vi "1.1.vi"() -> ()   [LabVIEW 2020]
panel:
  in  "MODO 6":bool
  out "6":bool
  in  "MODO 5":bool
  out "5":bool
  in  "MODO 4":bool
  out "4":bool
  in  "MODO 3":bool
  out "3":bool
  in  "MODO 2":bool
  out "2":bool
  in  "MODO 1":bool
  out "1":bool
  # "SWITCH WHEN PRESSED: ESTE MODO MECANICO CAMBIA DE VALORA CADA QUE\nES PRESIONADO"
  # "SWITCH WHEN RELEASED: ESTE MODO CAMBIA CUANDO SE DEJA DE PRESIONAR"
  # "SWITCH UNTIL RELEASEDESTE MODO CAMBIA CUANDO SE PRESIONA Y CUANDO SE \nDEJA DE PRESIONAR"
  # "LATCHES WHEN PRESSED: ESTE MODO CAMBIA DE VALOR CUANDO ES PRESIONADO Y \nRETIENE EL VALOR HASTA QUE EL INSTURMENTO VIRTUAL LO LEE, PUEDE USARSE COMO \nUN CONTADOR"
  # "LATCHES WHEN RELEASED:  ESTE MODO CAMBIA DE VALOR CUANDO SE DEJA DE \nPRESIONAR Y RETIENE EL VALOR HASTA QUE EL INSTURMENTO VIRTUAL LO LEE, \nPUEDE USARSE COMO UN CONTADOR"
  # "LATCHES UNTIL RELEASED:  ESTE MODO CAMBIA DE VALOR CUANDO ES PRESIONADO \nY TAMBIEN CUANDO SE DEJA DE PRESIONAR, RETIENE EL VALOR CUANDO PASA UNA DE \nESTAS DOS ACCIONES HASTA QUE EL INSTURMENTO VIRTUAL LO LEE, PUEDE USARSE \nCOMO UN CONTADOR"
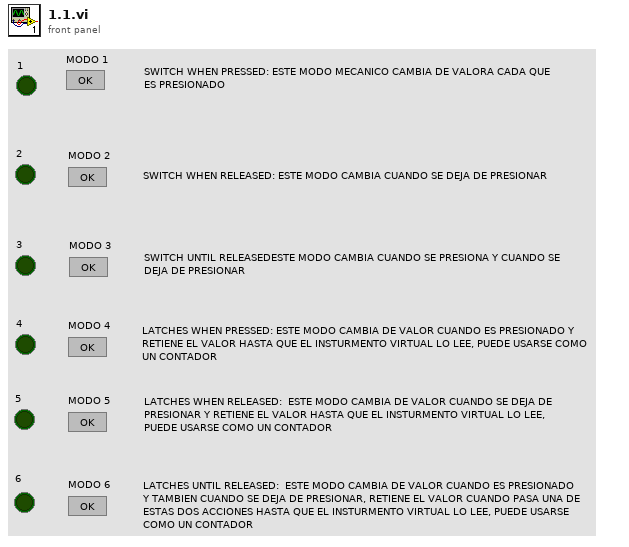
[diagram p1: front panel]
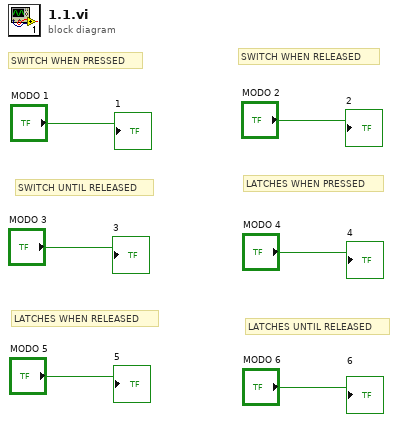
[diagram p0: block diagram]
diagram:
  # "LATCHES UNTIL RELEASED"
  # "LATCHES WHEN RELEASED"
  # "LATCHES WHEN PRESSED"
  # "SWITCH UNTIL RELEASED"
  # "SWITCH WHEN RELEASED"
  # "SWITCH WHEN PRESSED"
  "1" <- "MODO 1"
  "2" <- "MODO 2"
  "3" <- "MODO 3"
  "4" <- "MODO 4"
  "5" <- "MODO 5"
  "6" <- "MODO 6"
